vi "STM32BootLoader.vi"() -> ()   [LabVIEW 2018]
uses:
  <vilib>/Utility/file.llb/Read Delimited Spreadsheet (string).vi
  <vilib>/Instr/_visa.llb/VISA Configure Serial Port (Instr).vi
panel:
  out "elapsed time(S)":dbl
  out "millisecond timer value":u32
  out "start":bool=TRUE
  out "size(s)":i32
  out "index":i32
  out "Array":string[](array[string])
  in  "stop 2":bool
  out "ConnectStatus":bool
  in  "parity":enum16{"None", "Odd", "Even", "Mark", "Space"}(ring)
  in  "data bits":u16=8 min=5 max=8 step=1
  in  "baud rate":u32=9600
  in  "ComPort":refnum<visa-resource-name>
  in  "Connect":bool
  in  "Path":path
  in  "Program":bool
  in  "stop":bool
  out "Slide":u8(slide) scale=0.0..100.0
  out "MSG":string
  # "STM32 BOOTLOADER V1.0.0"
  # "Step1:Load App Hex File\nStep2:Connect Serial Port\nStep3:Click \"Program\"Button"
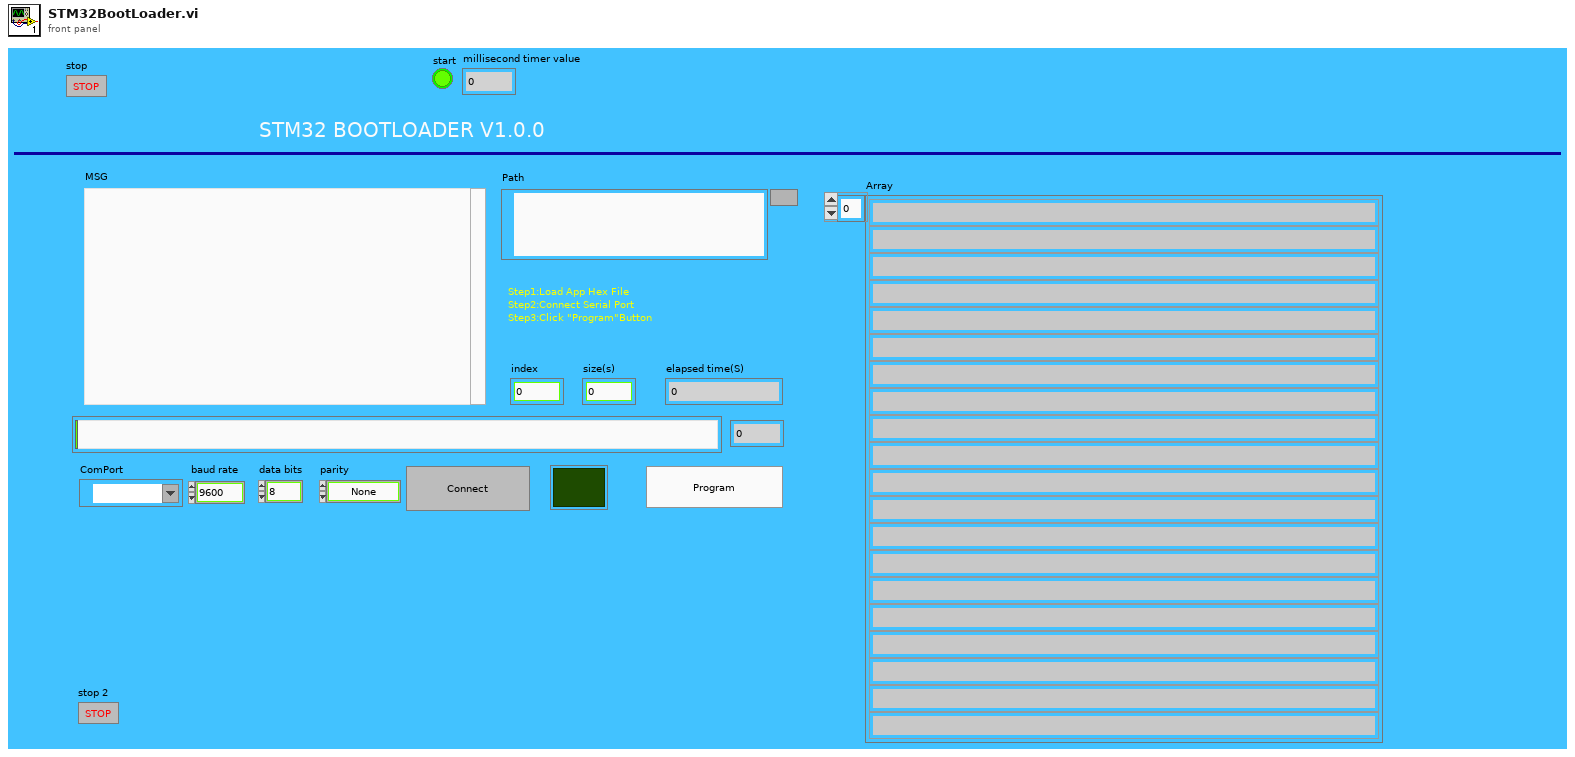
[diagram p1: front panel]
types:
  T1 = enum16{"EnterBootLoder", "StartToUpdate", "JumpToApp"}
  T2 = enum16{"EnterBootMode", "StartToProgram", "ProgramLineOK", "ProgramAllOk", "Error", "NULL"}
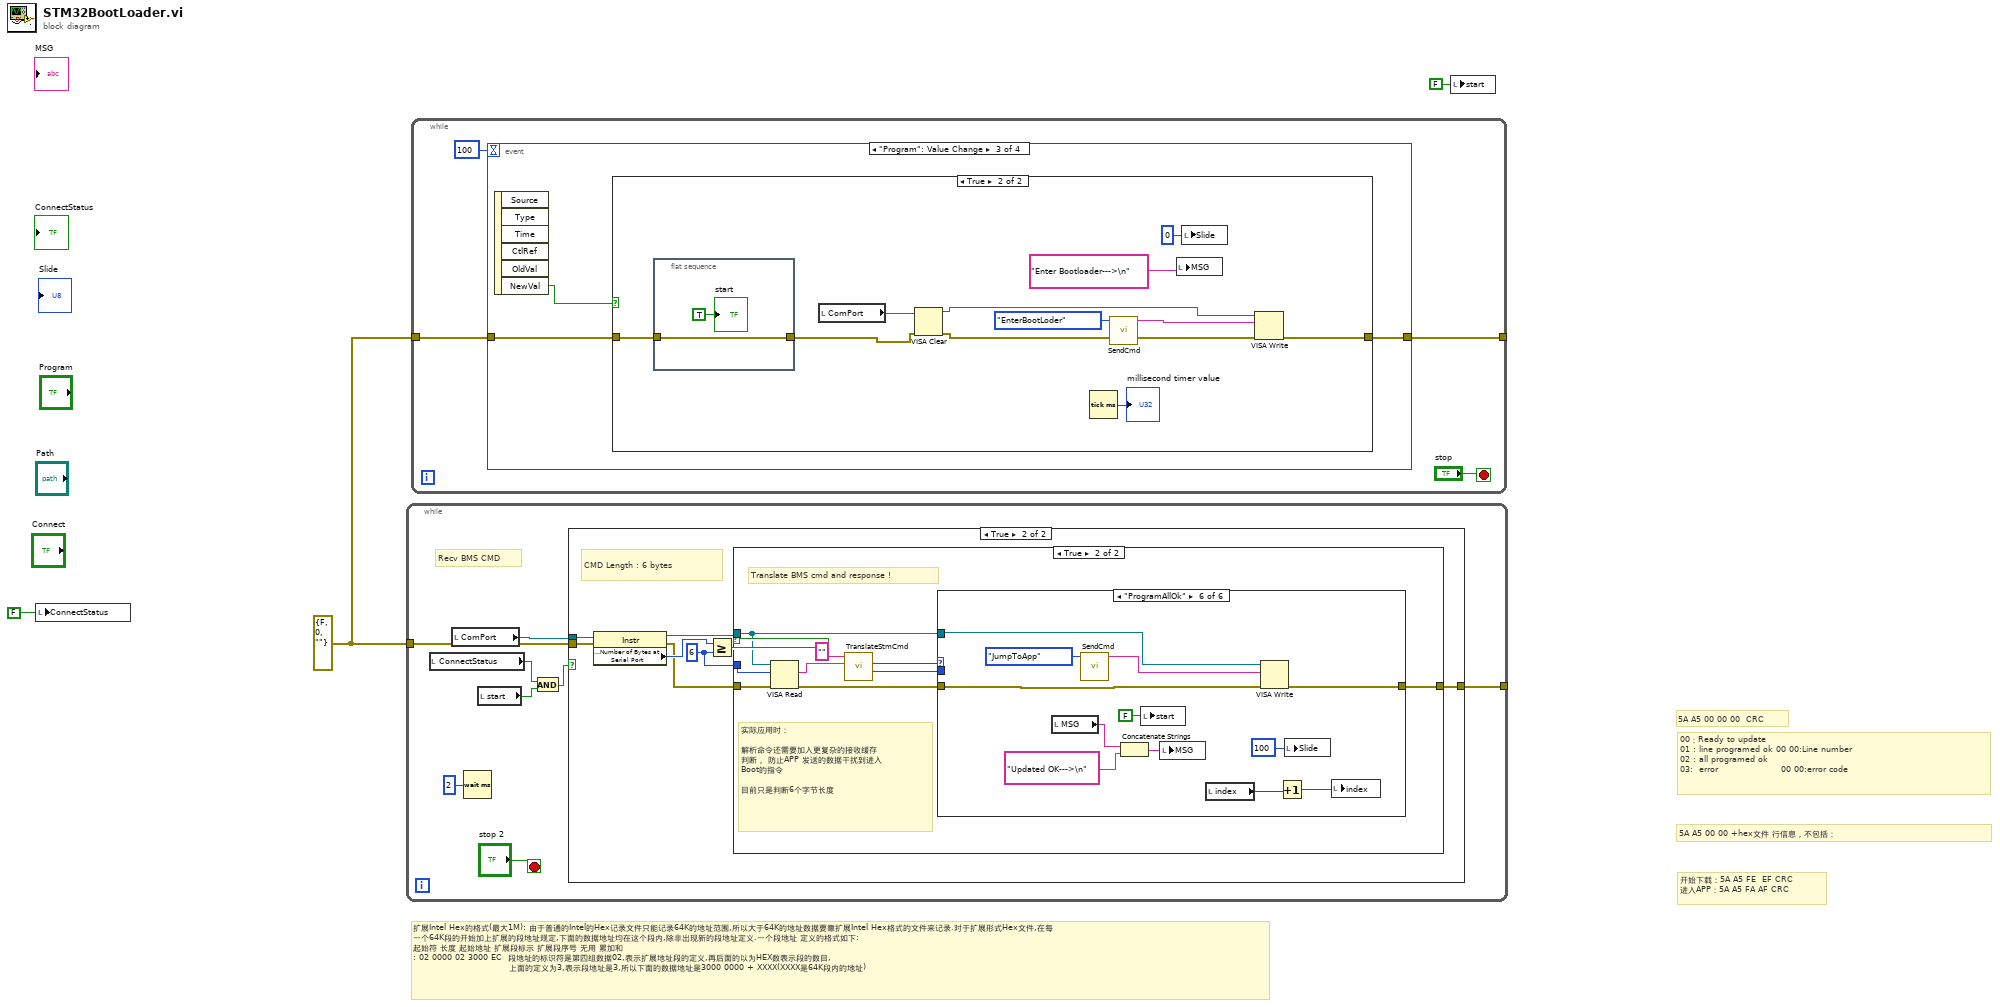
[diagram p0: block diagram]
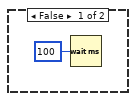
[diagram p2: hidden frame]
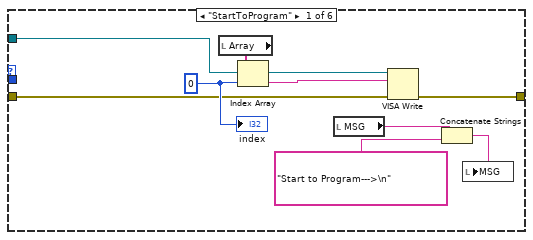
[diagram p4: hidden frame]
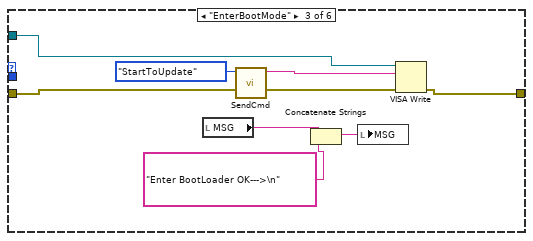
[diagram p6: hidden frame]
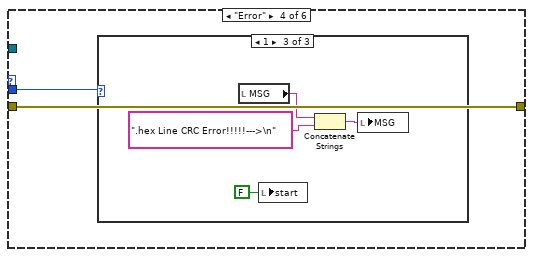
[diagram p7: hidden frame]
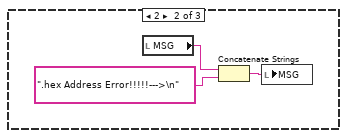
[diagram p9: hidden frame]
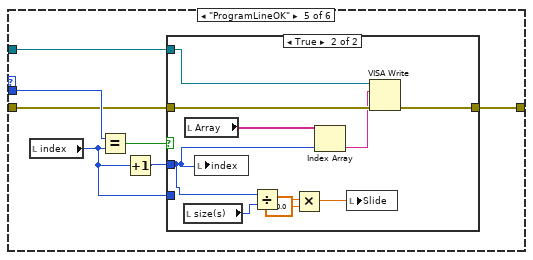
[diagram p10: hidden frame]
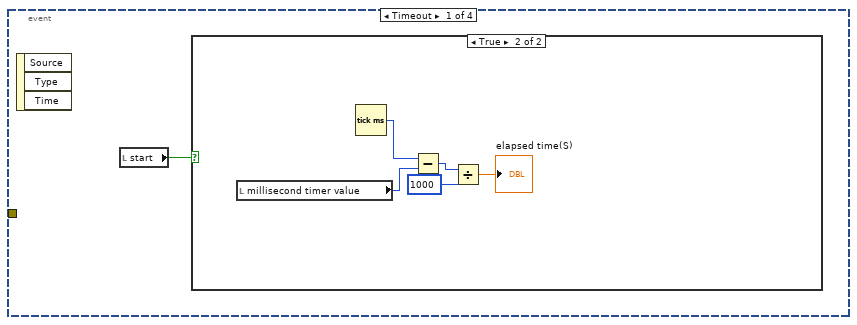
[diagram p12: hidden frame]
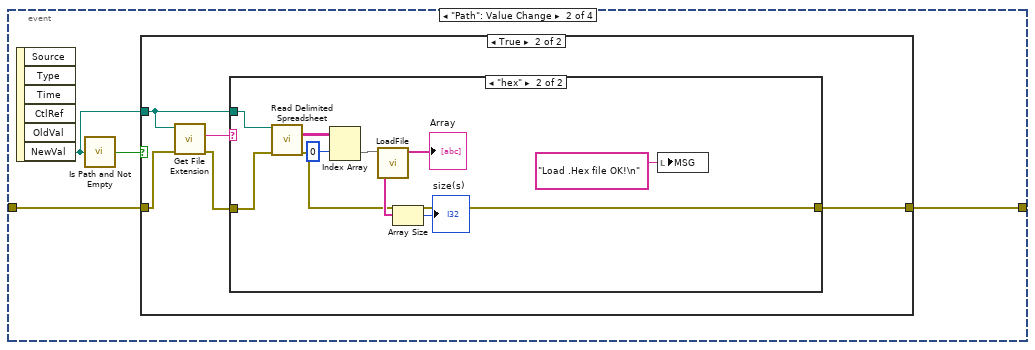
[diagram p14: hidden frame]
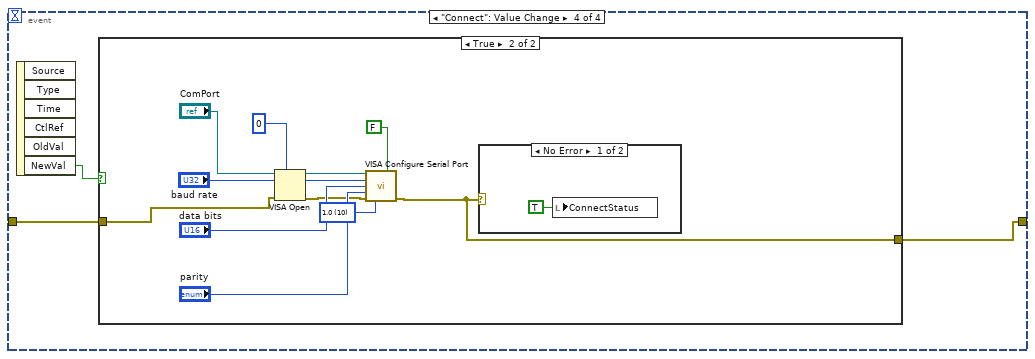
[diagram p18: hidden frame]
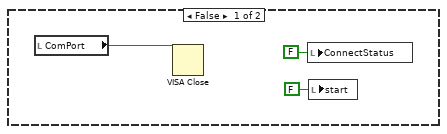
[diagram p19: hidden frame]
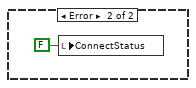
[diagram p20: hidden frame]
diagram:
  w2 = errorcluster {"status"=FALSE, "code"=0, "source"=""} ("error in (no error)")
  # "扩展Intel Hex的格式(最大1M): 由于普通的Intel的Hex记录文件只能记录64K的地址范围,所以大于64K的地址数据要靠扩展Intel Hex格式的文件来记录.对于扩展形式Hex文件,在每\n一个64K段的开始加上扩展的段地址规定,下面的数据地址均在这个段内,除非出现新的段地址定义.一个段地址 定义的格式如下:\n起始符 长度 起始地址 扩展段标示 扩展段序号 无用 累加和\n: 02 0000 02 3000 EC  段地址的标识符是第四组数据02,表示扩展地址段的定义,再后面的以为HEX数表示段的数目,\n                                上面的定义为3,表示段地址是3,所以下面的数据地址是3000 0000 + XXXX(XXXX是64K段内的地址)"
  # "开始下载：5A A5 FE  EF CRC\n进入APP：5A A5 FA AF CRC"
  # "5A A5 00 00 +hex文件 行信息，不包括："
  # "00：Ready to update    \n01 : line programed ok 00 00:Line number\n02 : all programed ok   \n03:  error                     00 00:error code"
  # "5A A5 00 00 00  CRC"
  n1 = local write "ConnectStatus"(FALSE ("ConnectStatus")) -> ()
  n2 = while {
    tunnel: w2 -> [w8]
    tunnel: [w7] -> _
    stop <- "stop 2" stop-if-true
    # "Recv BMS CMD"
    n3 = local read "ConnectStatus"() -> (w6:bool)
    n4 = local read "ComPort"() -> (w9:refnum<visa-resource-name>)
    n5 = Wait (ms)(milliseconds to wait=u32 2) -> ()  [unwired: 1 out]
    n6 = local read "start"() -> (w5:bool)
    n7 = And(x=w6, y=w5) -> (x .and. y?=w4:bool)
    n8 = case shown="True" w4 {
      tunnel: w9 -> [_ w16]
      tunnel: w8 -> [_ w15]
      tunnel: [_ w13] -> w7
      frame False {
        n9 = Wait (ms)(milliseconds to wait=u32 100) -> ()  [unwired: 1 out]
      }
      frame True {
        w17 = u8 6 ("y")
        # "CMD Length : 6 bytes"
        n10 = property class="Instr"(reference=w16, error in=w15) -> (reference out=w20:refnum<visa-resource-name>, error out=w14:errorcluster, "Serial Settings:Number of Bytes at Serial Port"=w19:u32)
        n11 = Greater Or Equal?(x=w19, y=w17) -> (x >= y?=w18:bool)
        n12 = case shown="True" w18 {
          tunnel: w20 -> [_ w25]
          tunnel: w17 -> [_ w27]
          tunnel: w14 -> [_ w24]
          tunnel: [_ w23] -> w13
          frame False {
          }
          frame True {
            # "实际应用时：\n\n解析命令还需要加入更复杂的接收缓存\n判断， 防止APP 发送的数据干扰到进入\nBoot的指令\n\n目前只是判断6个字节长度"
            # "Translate BMS cmd and response !"
            n13 = VISA Read(VISA resource name=w25, byte count=w27, error in (no error)=w24) -> (read buffer=w21:string, error out=w22:errorcluster)  [unwired: 2 out]
            n14 = call "TranslateStmCmd.vi"("String"=w21, "Buffer"="") -> ("數值"=w28:u16, "î‘B"=w29:T2)  [unwired: 8 in]
            n15 = case shown="\"ProgramAllOk\"" w29 {
              tunnel: w28 -> [_ _ _ w47 w62 _]
              tunnel: w25 -> [w33 _ w45 _ w58 w80]
              tunnel: [w31 _ w43 w48 w56 w78] -> w23
              tunnel: w22 -> [w32 _ w44 w48 w57 w79]
              frame "StartToProgram" {
                w38 = 0 ("index")
                n16 = local read "Array"() -> (w37:string[])
                n17 = Index Array(array=w37, index=w38) -> (element=w30:string)
                n18 = local read "MSG"() -> (w35:string)
                n19 = VISA Write(VISA resource name=w33, write buffer=w30, error in (no error)=w32) -> (error out=w31:errorcluster)  [unwired: 2 out]
                n20 = Concatenate Strings(w35, "Start to Program--->\n" ("MSG")) -> (w36:string)
                n21 = local write "MSG"(w36) -> ()
                "index" <- w38
              }
              frame "NULL", Default {
              }
              frame "EnterBootMode" {
                n22 = local read "MSG"() -> (w42:string)
                n23 = call "SendCmd.vi"("Function"=T1."StartToUpdate") -> ("concatenated string"=w39:string)  [unwired: 10 in]
                n24 = Concatenate Strings(w42, "Enter BootLoader OK--->\n" ("MSG")) -> (w40:string)
                n25 = local write "MSG"(w40) -> ()
                n26 = VISA Write(VISA resource name=w45, write buffer=w39, error in (no error)=w44) -> (error out=w43:errorcluster)  [unwired: 2 out]
              }
              frame "Error" {
                n27 = case shown="1" w47 {
                  frame 0, Default {
                  }
                  frame 2 {
                    n28 = local read "MSG"() -> (w50:string)
                    n29 = Concatenate Strings(w50, ".hex Address Error!!!!!--->\n" ("MSG")) -> (w51:string)
                    n30 = local write "MSG"(w51) -> ()
                  }
                  frame 1 {
                    n31 = local read "MSG"() -> (w54:string)
                    n32 = local write "start"(FALSE ("start")) -> ()
                    n33 = Concatenate Strings(w54, ".hex Line CRC Error!!!!!--->\n" ("MSG")) -> (w55:string)
                    n34 = local write "MSG"(w55) -> ()
                  }
                }
              }
              frame "ProgramLineOK" {
                n35 = local read "index"() -> (w59:i32)
                n36 = Equal?(x=w62, y=w59) -> (x = y?=w61:bool)
                n37 = Increment(x=w59) -> (x+1=w60:i32)
                n38 = case shown="True" w61 {
                  tunnel: w60 -> [_ w68]
                  tunnel: w59 -> [_ _]
                  tunnel: w58 -> [_ w71]
                  tunnel: w57 -> [_ w70]
                  tunnel: [_ w69] -> w56
                  frame False {
                  }
                  frame True {
                    n39 = local read "size(s)"() -> (w67:i32)
                    n40 = local read "Array"() -> (w72:string[])
                    n41 = local write "index"(w68) -> ()
                    n42 = Divide(x=w68, y=w67) -> (x/y=w66:dbl)
                    n43 = Multiply(x=w66, y=100.0) -> (x*y=w64:dbl)
                    n44 = Index Array(array=w72, index=w68) -> (element=w63:string)
                    n45 = local write "Slide"(w64) -> ()
                    n46 = VISA Write(VISA resource name=w71, write buffer=w63, error in (no error)=w70) -> (error out=w69:errorcluster)  [unwired: 2 out]
                  }
                }
              }
              frame "ProgramAllOk" {
                n47 = local read "MSG"() -> (w82:string)
                n48 = call "SendCmd.vi"("Function"=T1."JumpToApp") -> ("concatenated string"=w74:string)  [unwired: 10 in]
                n49 = Concatenate Strings(w82, "Updated OK--->\n" ("MSG")) -> (w83:string)
                n50 = local write "start"(FALSE ("start")) -> ()
                n51 = local write "MSG"(w83) -> ()
                n52 = local read "index"() -> (w76:i32)
                n53 = VISA Write(VISA resource name=w80, write buffer=w74, error in (no error)=w79) -> (error out=w78:errorcluster)  [unwired: 2 out]
                n54 = Increment(x=w76) -> (x+1=w77:i32)
                n55 = local write "Slide"(u8 100 ("Slide")) -> ()
                n56 = local write "index"(w77) -> ()
              }
            }
          }
        }
      }
    }
  }
  n57 = while {
    tunnel: w2 -> [w87]
    tunnel: [w86] -> _
    stop <- "stop" stop-if-true
    n58 = event shown="[2] \"Program\": Value Change" {
      selector: _ -> [_ _ _ _]
      dyn-events: _ -> [_ _ _ _]
      timeout: 100 -> [_ _ _ _]
      tunnel: w87 -> [_ w96 w114 w130]
      tunnel: [_ w95 w113 w129] -> w86
      event Timeout {
        n59 = event-data() -> ()  [unwired: 1 in, 3 out]
        n60 = local read "start"() -> (w89:bool)
        n61 = case shown="True" w89 {
          frame False {
          }
          frame True {
            n62 = local read "millisecond timer value"() -> (w93:u32)
            n63 = Tick Count (ms)() -> (millisecond timer value=w94:u32)
            n64 = Subtract(x=w94, y=w93) -> (x-y=w92:u32)
            n65 = Divide(x=w92, y=u32 1000) -> (x/y=→"elapsed time(S)":dbl)
          }
        }
      }
      event "Path": Value Change {
        n66 = event-data() -> ("NewVal"=w97:path)  [unwired: 1 in, 5 out]
        n67 = call <vilib>:"Is Path and Not Empty.vi"("path"=w97) -> ("Is Path and Not Empty?"=w98:bool)  [unwired: 4 in]
        n68 = case shown="True" w98 {
          tunnel: w97 -> [_ w102]
          tunnel: w96 -> [_ w101]
          tunnel: [_ w99] -> w95
          frame False {
          }
          frame True {
            n69 = call <vilib>:"Get File Extension.vi"("error in (no error)"=w101, "file"=w102) -> ("error out"=w100:errorcluster, "lowercase file extension"=w103:string)  [unwired: 5 in, 3 out]
            n70 = case shown="\"hex\"" w103 {
              tunnel: w102 -> [_ w112]
              tunnel: w100 -> [_ w105]
              tunnel: [_ w104] -> w99
              frame "False", Default {
              }
              frame "hex" {
                n71 = call-poly <vilib>:"Read Delimited Spreadsheet.vi"("file path (dialog if empty)"=w112, "error in (no error)"=w105) -> ("all rows"=w111:string[][], "error out"=w104:errorcluster)  [unwired: 8 in, 4 out]
                n72 = Index Array(array=w111, index (col)=0 ("disabled index (col)")) -> (element=w109:string[])  [unwired: 1 in]
                n73 = call "LoadFile.vi"("all rows"=w109) -> ("Array"=w108:string[])  [unwired: 10 in]
                "Array" <- w108
                n74 = Array Size(array=w108) -> (size(s)=→"size(s)":i32)
                n75 = local write "MSG"("Load .Hex file OK!\n" ("MSG")) -> ()
              }
            }
          }
        }
      }
      event "Program": Value Change {
        n76 = event-data() -> ("NewVal"=w115:bool)  [unwired: 1 in, 5 out]
        n77 = case shown="True" w115 {
          tunnel: w114 -> [_ w116]
          tunnel: [_ w124] -> w113
          frame False {
          }
          frame True {
            n78 = flat-sequence {
              tunnel: [w127] -> w117
              tunnel: w116 -> [w127]
              frame #0 {
                "start" <- TRUE
              }
            }
            n79 = local read "ComPort"() -> (w123:refnum<visa-resource-name>)
            n80 = VISA Clear(VISA resource name=w123, error in (no error)=w117) -> (VISA resource name out=w122:refnum<visa-resource-name>, error out=w121:errorcluster)
            n81 = Tick Count (ms)() -> (millisecond timer value=→"millisecond timer value":u32)
            n82 = call "SendCmd.vi"("Function"=T1."EnterBootLoder") -> ("concatenated string"=w119:string)  [unwired: 10 in]
            n83 = local write "MSG"("Enter Bootloader--->\n" ("MSG")) -> ()
            n84 = local write "Slide"(u8 0 ("Slide")) -> ()
            n85 = VISA Write(VISA resource name=w122, write buffer=w119, error in (no error)=w121) -> (error out=w124:errorcluster)  [unwired: 2 out]
          }
        }
      }
      event "Connect": Value Change {
        n86 = event-data() -> ("NewVal"=w131:bool)  [unwired: 1 in, 5 out]
        n87 = case shown="True" w131 {
          tunnel: w130 -> [_ w137]
          tunnel: [_ w135] -> w129
          frame False {
            n88 = local read "ComPort"() -> (w134:refnum<visa-resource-name>)
            n89 = VISA Close(VISA resource name=w134) -> ()  [unwired: 1 in, 1 out]
            n90 = local write "ConnectStatus"(FALSE ("ConnectStatus")) -> ()
            n91 = local write "start"(FALSE ("start")) -> ()
          }
          frame True {
            w138 = u16 10 items=["1.0"=10, "1.5"=15, "2.0"=20] ("stop bits (10: 1 bit)")
            n92 = VISA Open(timeout (0)=u32 0 ("VISA Open timeout (0)"), error in (no error)=w137, VISA resource name="ComPort") -> (VISA resource name=w144:refnum<visa-resource-name>, error out=w136:errorcluster)  [unwired: 2 in]
            n93 = call-poly "VISA Configure Serial Port"("VISA resource name"=w144, "Enable Termination\nChar (T)"=FALSE ("Enable Termination\nChar (T)"), "baud rate (9600)"="baud rate", "data bits (8)"="data bits", "parity (0:none)"="parity", "error in (no error)"=w136, "stop bits (10: 1 bit)"=w138) -> ("error out"=w135:errorcluster)  [unwired: 7 in, 1 out]
            n94 = case shown="No Error" w135 {
              frame No Error {
                n95 = local write "ConnectStatus"(TRUE ("ConnectStatus")) -> ()
              }
              frame Error {
                n96 = local write "ConnectStatus"(FALSE ("ConnectStatus")) -> ()
              }
            }
          }
        }
      }
    }
  }
  n97 = local write "start"(FALSE ("start")) -> ()
